vi "start.vi"(8 "error in (no error)":errorcluster, 11 "FPGAWrapperAN110607Galvo in":refnum<class "FPGAWrapperAN110607Galvo.lvclass">) -> (0 "error out":errorcluster, 3 "FPGAWrapperAN110607Galvo out":refnum<class "FPGAWrapperAN110607Galvo.lvclass">)   [LabVIEW 2010, in "FPGAWrapperAN110607Galvo.lvclass"]
uses:
  FPGAWrapperAN110607Galvo.lvclass
  <vilib>/rvi/interface/nirviReadWriteControl/nirviReadWriteControl.xnode
  FPGA_VI_ref.ctl
  <vilib>/rvi/interface/common/niFpgaNodeNameForErrorReporting.ctl
  <vilib>/rvi/errors/niLvFpgaWhatHappensToTopLevelVI.ctl
  <vilib>/Utility/error.llb/Error Cluster From Error Code.vi
  <vilib>/rvi/errors/niLvFpgaAdjustHostInterfaceError.vi
  NiFpgaLv.dll
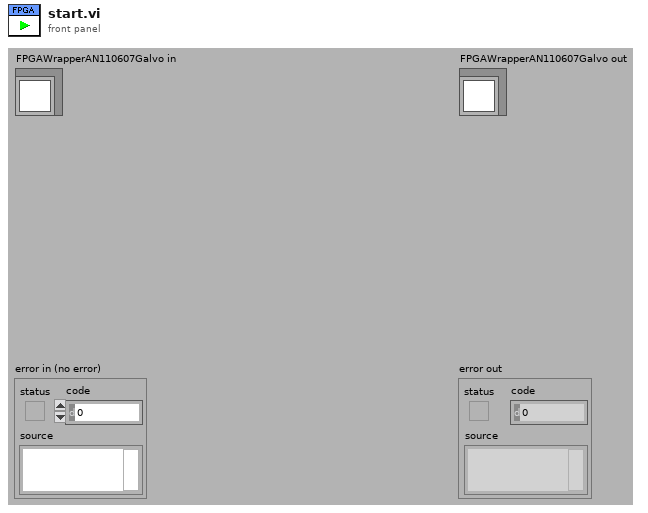
[diagram p1: front panel]
types:
  T1 = typedef "niFpgaNodeNameForErrorReporting.ctl" = enum16{"Open FPGA VI Reference", "Read/Write Control", "Invoke Method: Abort", "Invoke Method: Acknowledge IRQ", "Invoke Method: Download", "Invoke Method: FIFO.Configure", "Invoke Method: FIFO.Read", "Invoke Method: FIFO.Start", "Invoke Method: FIFO.Stop", "Invoke Method: FIFO.Write", "Invoke Method: Reset", "Invoke Method: Run", "Invoke Method: Wait on IRQ", "Close FPGA VI Reference"}
  T2 = typedef "niLvFpgaWhatHappensToTopLevelVI.ctl" = enum16{"top level VI scripted behind XNode", "top level VI inlined behind XNode"}
  T3 = typedef "FPGAWrapperAN110607Galvo.lvclass/FPGA_VI_ref.ctl" = refnum<k20>
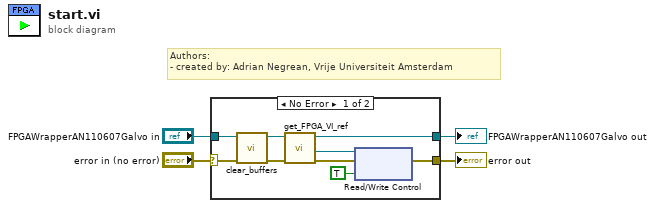
[diagram p0: block diagram]
diagram:
  # "Authors: \n- created by: Adrian Negrean, Vrije Universiteit Amsterdam"
  n1 = case shown="No Error" "error in (no error)" {
    selector: "error in (no error)" -> [w6 w53]
    tunnel: [w11 w53] -> w3
    tunnel: "FPGAWrapperAN110607Galvo in" -> [w8 w54]
    tunnel: [w9 w54] -> w1
    frame No Error {
      n2 = call-dynamic "clear_buffers.vi"("error in (no error)"=w6, "FPGAWrapperAN110607Galvo in"=w8) -> ("error out"=w5:errorcluster, "FPGAWrapperAN110607Galvo out"=w7:refnum<class "FPGAWrapperAN110607Galvo.lvclass">)  [unwired: 8 in]
      n3 = call-dynamic "get_FPGA_VI_ref.vi"("error in (no error)"=w5, "FPGAWrapperAN110607Galvo in"=w7) -> ("error out"=w12:errorcluster, "FPGA VI reference"=w13:T3, "FPGAWrapperAN110607Galvo out"=w9:refnum<class "FPGAWrapperAN110607Galvo.lvclass">)  [unwired: 6 in, 1 out]
      n4 = xnode "Read/Write Control"("FPGA VI Reference In"=w13, "error in"=w12, "acquire"=TRUE) -> ("error out"=w11:errorcluster)  [unwired: 1 out]
    }
    frame Error {
    }
  }
  "error out" <- w3
  "FPGAWrapperAN110607Galvo out" <- w1
